vi "Positions.vi"(6 "Limit switch 5":bool, 7 "Limit switch 4":bool, 8 "Limit switch 3":bool, 9 "Limit switch 2":bool, 11 "Positions":enum16{"0", "1", "2", "3", "4"}(ring)) -> ()   [LabVIEW 2014]
panel:
  in  "Limit switch 1":bool
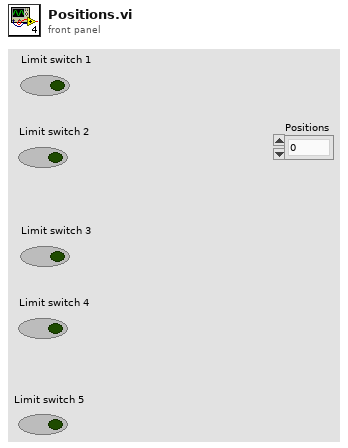
[diagram p1: front panel]
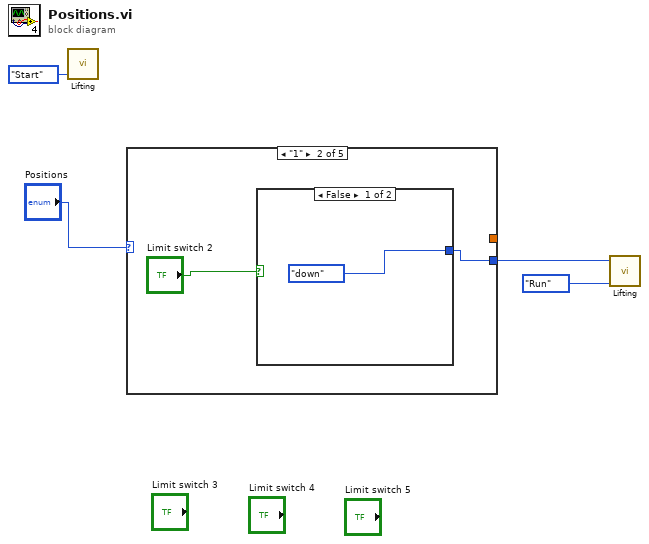
[diagram p0: block diagram]
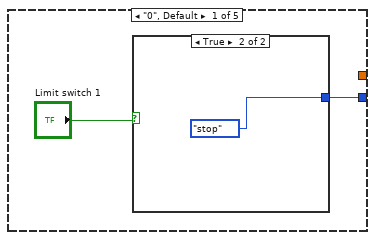
[diagram p2: hidden frame]
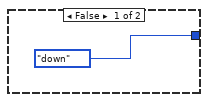
[diagram p3: hidden frame]
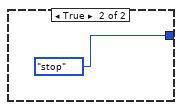
[diagram p4: hidden frame]
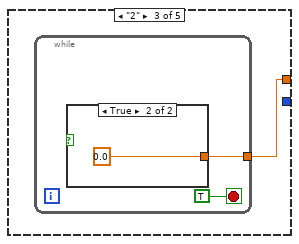
[diagram p5: hidden frame]
diagram:
  n1 = call "Lifting.vi"("Mode"=enum8{"Start", "Run", "Finish"}."Start") -> ()  [unwired: 5 in]
  n2 = case shown="\"1\"" "Positions" {
    tunnel: [_ _ w13 _ _] -> _
    tunnel: [w5 w9 _ _ _] -> w1
    frame "0", Default {
      n3 = case shown="True" "Limit switch 1" {
        tunnel: [enum16{"stop", "up", "down"}."down" ("Direction") enum16{"stop", "up", "down"}."stop" ("Direction")] -> w5
        frame False {
        }
        frame True {
        }
      }
    }
    frame "1" {
      n4 = case shown="False" "Limit switch 2" {
        tunnel: [enum16{"stop", "up", "down"}."down" ("Direction") enum16{"stop", "up", "down"}."stop" ("Direction")] -> w9
        frame False {
        }
        frame True {
        }
      }
    }
    frame "2" {
      n5 = while {
        tunnel: [w14] -> w13
        stop <- TRUE stop-if-true
        n6 = case shown="True" {
          selector: _ -> [_ _]
          tunnel: [_ 0.0 ("Motorspeed")] -> w14
          frame False {
          }
          frame True {
          }
        }
      }
    }
    frame "3" {
    }
    frame "4" {
    }
  }
  n7 = call "Lifting.vi"("Mode"=enum8{"Start", "Run", "Finish"}."Run", "Direction"=w1) -> ()  [unwired: 4 in]
